vi "Example.vi"() -> ()   [LabVIEW 2020]
uses:
  Example Sink/Example Sink/Example Sink.lvclass
  C:/Program Files/National Instruments/LabVIEW 2020/vi.lib/ActorFramework/Actor/Actor.lvclass
  Example Source/Example Source/Example Source.lvclass
  C:/Users/huipeng8/Desktop/Event-Source-Actor/Source/Using Template/Timed Loop Controller/Timed Loop Controller/Timed Loop Controller.lvclass
  Example logger/Example logger/Example logger.lvclass
  Source/Template Source/Event Source Messages/Unregister For Event Msg/Unregister For Event Msg.lvclass/Unregister For Event Msg.ctl
  <vilib>/ActorFramework/Message Enqueuer/Message Enqueuer.lvclass/Message Enqueuer.ctl
  Source/Template Source/Event Source Messages/Register For Event Msg/Register For Event Msg.lvclass/Register For Event Msg.ctl
  Source/Template Source/Event Source Messages/Unregister Msg/Unregister Msg.lvclass/Unregister Msg.ctl
  <vilib>/ActorFramework/Message Enqueuer/Enqueue.vi
  Source/Template Source/Event Source Messages/Unregister For Event Msg/Unregister For Event Msg.lvclass
  C:/Program Files/National Instruments/LabVIEW 2020/vi.lib/ActorFramework/Message/Message.lvclass
  Source/Template Source/Event Source Messages/Register For Event Msg/Register For Event Msg.lvclass
  Source/Template Source/Event Source Messages/Unregister Msg/Unregister Msg.lvclass
  <vilib>/ActorFramework/Stop Msg/Stop Msg.lvclass
  <vilib>/ActorFramework/Message Priority Queue/Priority Enqueue.vi
  Source/Using Template/Timed Loop Controller/Timed Loop Controller/Timed Loop Controller.lvclass
  <vilib>/ActorFramework/Actor/Actor.lvclass
panel:
  in  "data":bool
  in  "time":bool
  in  "stop":bool
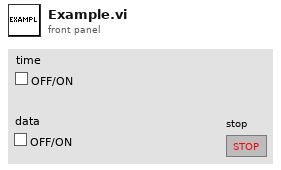
[diagram p1: front panel]
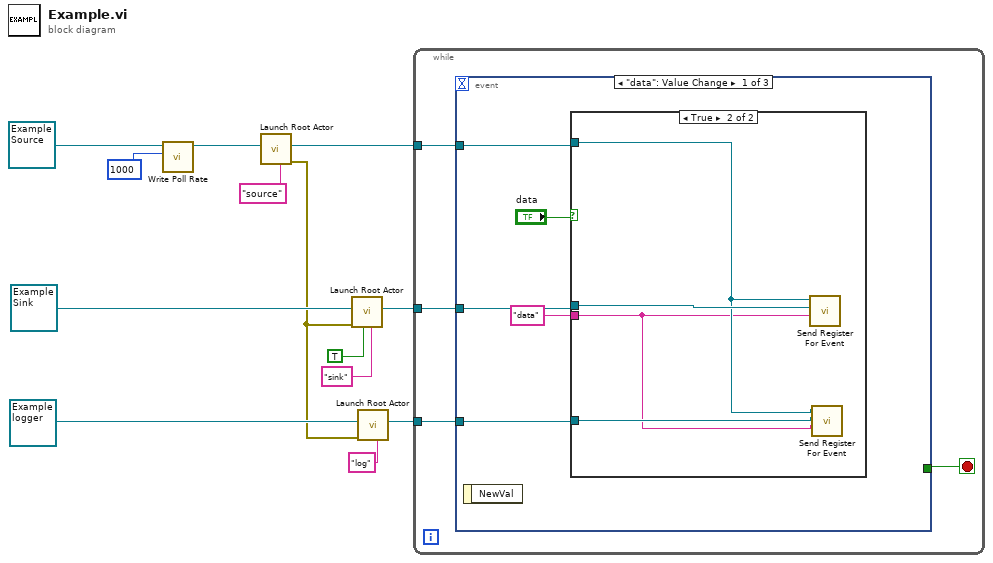
[diagram p0: block diagram]
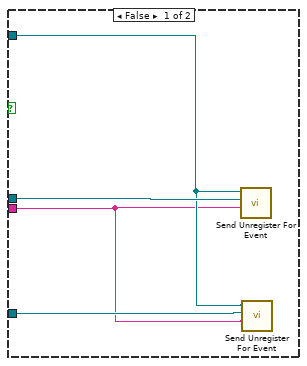
[diagram p2: hidden frame]
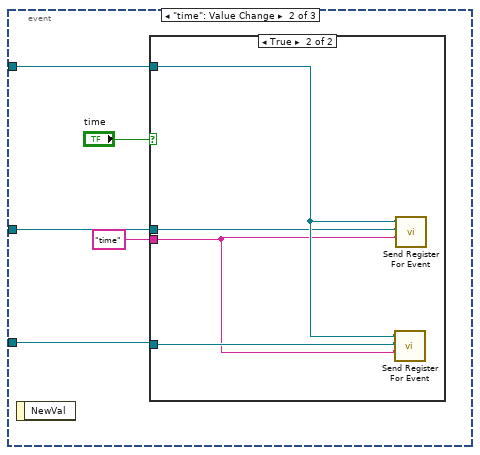
[diagram p3: hidden frame]
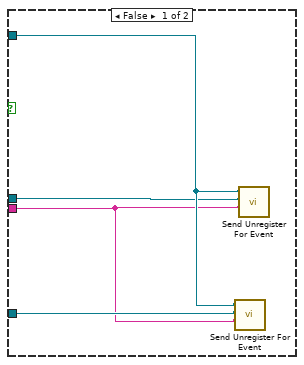
[diagram p4: hidden frame]
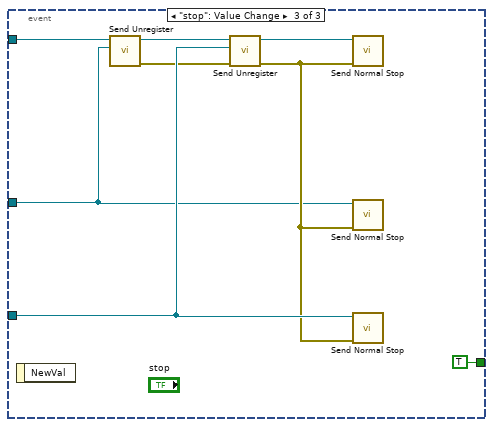
[diagram p5: hidden frame]
diagram:
  n1 = call "Write Poll Rate.vi"("Poll Rate"=u32 1000, "Timed Loop Controller in"=refnum<class "Example Source.lvclass"> refnum ("Example Source.lvlib:Example Source.lvclass")) -> ("Timed Loop Controller out"=w1:refnum<class "Example Source.lvclass">)  [unwired: 8 in, 1 out]
  n2 = call <vilib>:"Launch Root Actor.vi"("Debug Alias"="source", "Actor"=w1) -> ("error out"=w4:errorcluster, "Actor's Enqueuer"=w9:refnum<class "Message Enqueuer.lvclass">)  [unwired: 8 in]
  n3 = call <vilib>:"Launch Root Actor.vi"("Debug Alias"="sink", "Open Actor Core front panel? (F)"=TRUE, "error in (no error)"=w4, "Actor"=refnum<class "Example Sink.lvclass"> refnum ("Example Sink.lvlib:Example Sink.lvclass")) -> ("Actor's Enqueuer"=w7:refnum<class "Message Enqueuer.lvclass">)  [unwired: 6 in, 1 out]
  n4 = call <vilib>:"Launch Root Actor.vi"("Debug Alias"="log", "error in (no error)"=w4, "Actor"=refnum<class "Example logger.lvclass"> refnum ("Example logger.lvlib:Example logger.lvclass")) -> ("Actor's Enqueuer"=w2:refnum<class "Message Enqueuer.lvclass">)  [unwired: 7 in, 1 out]
  n5 = while {
    tunnel: w9 -> [w17]
    tunnel: w7 -> [w15]
    tunnel: w2 -> [w14]
    stop <- w16 stop-if-true
    n6 = event shown="[0] \"data\": Value Change" {
      selector: _ -> [_ _ _]
      dyn-events: _ -> [_ _ _]
      timeout: _ -> [_ _ _]
      tunnel: w17 -> [w22 w35 w46]
      tunnel: [_ _ TRUE ("stop")] -> w16
      tunnel: w15 -> [w21 w33 w47]
      tunnel: w14 -> [w20 w32 w50]
      event "data": Value Change {
        n7 = event-data() -> ()  [unwired: 1 in, 1 out]
        n8 = case shown="True" "data" {
          tunnel: w22 -> [w25 w29]
          tunnel: "data" ("Event Name") -> [w23 w27]
          tunnel: w21 -> [w26 w30]
          tunnel: w20 -> [w24 w28]
          frame False {
            n9 = call "Send Unregister For Event.vi"("Event Name"=w23, "Registrant Address"=w26, "Message Enqueuer"=w25) -> ()  [unwired: 7 in, 2 out]
            n10 = call "Send Unregister For Event.vi"("Event Name"=w23, "Registrant Address"=w24, "Message Enqueuer"=w25) -> ()  [unwired: 7 in, 2 out]
          }
          frame True {
            n11 = call "Send Register For Event.vi"("Event Name"=w27, "Registrant Enq"=w30, "Message Enqueuer"=w29) -> ()  [unwired: 7 in, 2 out]
            n12 = call "Send Register For Event.vi"("Event Name"=w27, "Registrant Enq"=w28, "Message Enqueuer"=w29) -> ()  [unwired: 7 in, 2 out]
          }
        }
      }
      event "time": Value Change {
        n13 = event-data() -> ()  [unwired: 1 in, 1 out]
        n14 = case shown="True" "time" {
          tunnel: w35 -> [w38 w42]
          tunnel: "time" ("Event Name") -> [w36 w40]
          tunnel: w33 -> [w37 w41]
          tunnel: w32 -> [w39 w43]
          frame False {
            n15 = call "Send Unregister For Event.vi"("Event Name"=w36, "Registrant Address"=w39, "Message Enqueuer"=w38) -> ()  [unwired: 7 in, 2 out]
            n16 = call "Send Unregister For Event.vi"("Event Name"=w36, "Registrant Address"=w37, "Message Enqueuer"=w38) -> ()  [unwired: 7 in, 2 out]
          }
          frame True {
            n17 = call "Send Register For Event.vi"("Event Name"=w40, "Registrant Enq"=w43, "Message Enqueuer"=w42) -> ()  [unwired: 7 in, 2 out]
            n18 = call "Send Register For Event.vi"("Event Name"=w40, "Registrant Enq"=w41, "Message Enqueuer"=w42) -> ()  [unwired: 7 in, 2 out]
          }
        }
      }
      event "stop": Value Change {
        n19 = event-data() -> ()  [unwired: 1 in, 1 out]
        n20 = call "Send Unregister.vi"("Registrant Enq"=w47, "Message Enqueuer"=w46) -> ("error out"=w44:errorcluster, "Message Enqueuer out"=w45:refnum<class "Message Enqueuer.lvclass">)  [unwired: 8 in]
        n21 = call "Send Unregister.vi"("error in"=w44, "Registrant Enq"=w50, "Message Enqueuer"=w45) -> ("error out"=w48:errorcluster, "Message Enqueuer out"=w49:refnum<class "Message Enqueuer.lvclass">)  [unwired: 7 in]
        n22 = call <vilib>:"Send Normal Stop.vi"("error in (no error)"=w48, "Message Enqueuer"=w49) -> ()  [unwired: 9 in, 1 out]
        n23 = call <vilib>:"Send Normal Stop.vi"("error in (no error)"=w48, "Message Enqueuer"=w47) -> ()  [unwired: 9 in, 1 out]
        n24 = call <vilib>:"Send Normal Stop.vi"("error in (no error)"=w48, "Message Enqueuer"=w50) -> ()  [unwired: 9 in, 1 out]
      }
    }
  }
